vi "delay.vi"(10 "String":string, 11 "String 2":string) -> (1 "Delay calculé":string)   [LabVIEW 2020]
panel:
  # "28/09/2023_14:08:36\n28/09/2023_14:08:36"
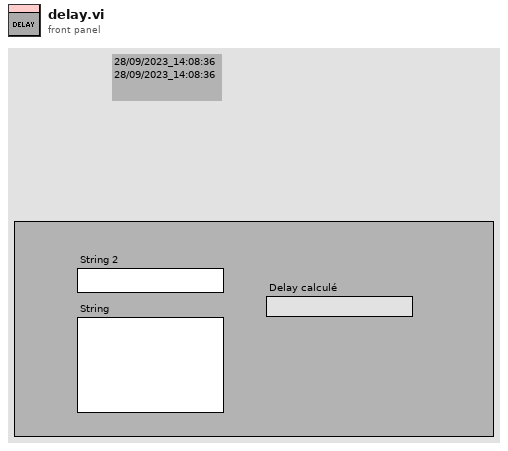
[diagram p1: front panel]
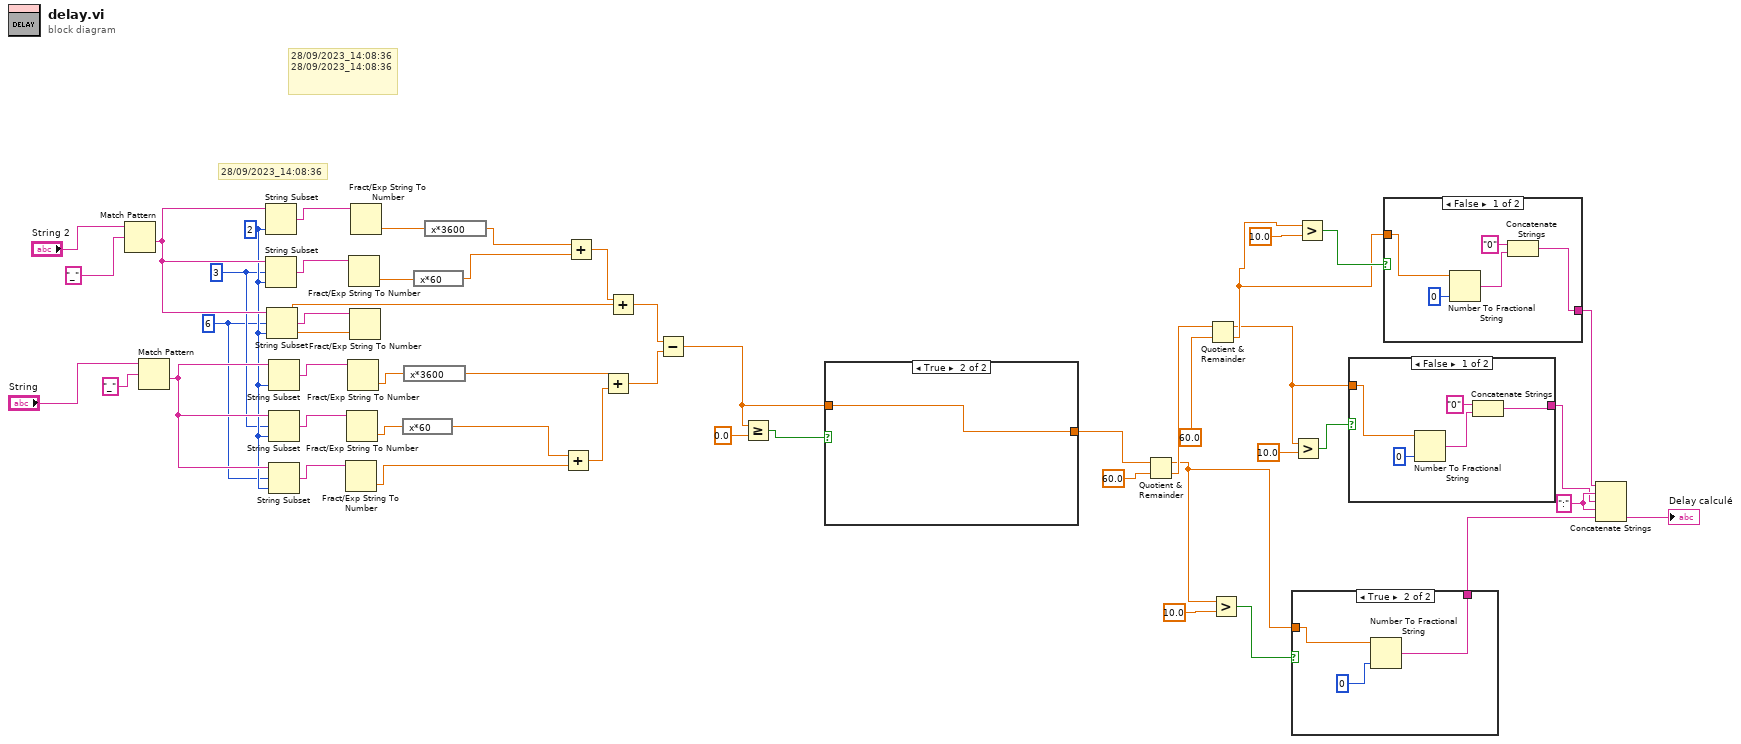
[diagram p0: block diagram]
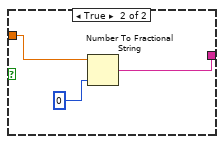
[diagram p2: hidden frame]
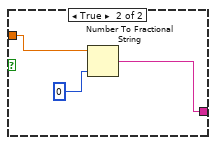
[diagram p3: hidden frame]
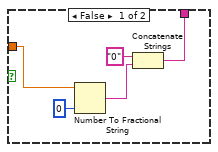
[diagram p4: hidden frame]
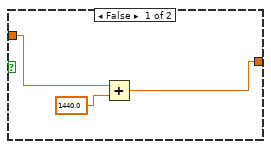
[diagram p5: hidden frame]
diagram:
  w16 = ":" ("string")
  w42 = 6 ("offset (0)")
  w43 = 3 ("offset (0)")
  w44 = 2 ("length (rest)")
  # "28/09/2023_14:08:36"
  # "28/09/2023_14:08:36\n28/09/2023_14:08:36"
  n1 = Match Pattern(string="String 2", regular expression="_") -> (after substring=w46:string)  [unwired: 1 in, 3 out]
  n2 = Match Pattern(string="String", regular expression="_") -> (after substring=w45:string)  [unwired: 1 in, 3 out]
  n3 = String Subset(string=w46, length (rest)=w44) -> (substring=w41:string)  [unwired: 1 in]
  n4 = String Subset(string=w46, offset (0)=w43, length (rest)=w44) -> (substring=w40:string)
  n5 = String Subset(string=w46, offset (0)=w42, length (rest)=w44) -> (substring=w39:string)
  n6 = String Subset(string=w45, length (rest)=w44) -> (substring=w38:string)  [unwired: 1 in]
  n7 = String Subset(string=w45, offset (0)=w43, length (rest)=w44) -> (substring=w37:string)
  n8 = String Subset(string=w45, offset (0)=w42, length (rest)=w44) -> (substring=w36:string)
  n9 = Fract/Exp String To Number(string=w36) -> (number=w27:dbl)  [unwired: 3 in, 1 out]
  n10 = Fract/Exp String To Number(string=w37) -> (number=w33:dbl)  [unwired: 3 in, 1 out]
  n11 = Fract/Exp String To Number(string=w38) -> (number=w32:dbl)  [unwired: 3 in, 1 out]
  n12 = Fract/Exp String To Number(string=w40) -> (number=w34:dbl)  [unwired: 3 in, 1 out]
  n13 = Fract/Exp String To Number(string=w39) -> (number=w29:dbl)  [unwired: 3 in, 1 out]
  n14 = Fract/Exp String To Number(string=w41) -> (number=w35:dbl)  [unwired: 3 in, 1 out]
  n15 = expression code="x*60"(w33) -> (w26:dbl)
  n16 = expression code="x*3600"(w32) -> (w25:dbl)
  n17 = expression code="x*60"(w34) -> (w30:dbl)
  n18 = expression code="x*3600"(w35) -> (w31:dbl)
  n19 = Add(x=w26, y=w27) -> (x+y=w24:dbl)
  n20 = Add(x=w31, y=w30) -> (x+y=w28:dbl)
  n21 = Add(x=w25, y=w24) -> (x+y=w22:dbl)
  n22 = Add(x=w28, y=w29) -> (x+y=w23:dbl)
  n23 = Subtract(x=w23, y=w22) -> (x-y=w19:dbl)
  n24 = Greater Or Equal?(x=w19, y=0.0) -> (x >= y?=w20:bool)
  n25 = case shown="True" w20 {
    tunnel: w19 -> [w53 w54]
    tunnel: [w52 w54] -> w13
    frame False {
      n26 = Add(x=w53, y=1440.0) -> (x+y=w52:dbl)
    }
    frame True {
    }
  }
  n27 = Quotient & Remainder(x=w13, y=60.0) -> (x-y*floor(x/y)=w10:dbl, floor(x/y)=w14:dbl)
  n28 = Quotient & Remainder(x=w14, y=60.0) -> (x-y*floor(x/y)=w2:dbl, floor(x/y)=w6:dbl)
  n29 = Greater?(x=w10, y=10.0) -> (0:w11:bool)
  n30 = case shown="True" w11 {
    tunnel: w10 -> [w59 w62]
    tunnel: [w56 w61] -> w9
    frame False {
      n31 = Number To Fractional String(number=w59, precision (6)=i16 0) -> (F-format string=w57:string)  [unwired: 2 in]
      n32 = Concatenate Strings("0" ("string"), w57) -> (w56:string)
    }
    frame True {
      n33 = Number To Fractional String(number=w62, precision (6)=i16 0) -> (F-format string=w61:string)  [unwired: 2 in]
    }
  }
  n34 = Greater?(x=w2, y=10.0) -> (0:w3:bool)
  n35 = Greater?(x=w6, y=10.0) -> (0:w7:bool)
  n36 = case shown="False" w3 {
    tunnel: [w65 w70] -> w1
    tunnel: w2 -> [w64 w68]
    frame False {
      n37 = Number To Fractional String(number=w64, precision (6)=i16 0) -> (F-format string=w66:string)  [unwired: 2 in]
      n38 = Concatenate Strings("0" ("string"), w66) -> (w65:string)
    }
    frame True {
      n39 = Number To Fractional String(number=w68, precision (6)=i16 0) -> (F-format string=w70:string)  [unwired: 2 in]
    }
  }
  n40 = case shown="False" w7 {
    tunnel: w6 -> [w75 w78]
    tunnel: [w72 w76] -> w5
    frame False {
      n41 = Number To Fractional String(number=w75, precision (6)=i16 0) -> (F-format string=w73:string)  [unwired: 2 in]
      n42 = Concatenate Strings("0" ("string"), w73) -> (w72:string)
    }
    frame True {
      n43 = Number To Fractional String(number=w78, precision (6)=i16 0) -> (F-format string=w76:string)  [unwired: 2 in]
    }
  }
  n44 = Concatenate Strings(w5, w16, w1, w16, w9) -> (→"Delay calculé":string)
